vi "get_level.vi"(8 "error in (no error)":errorcluster, 11 "File Log Provider in":refnum<class "File Log Provider.lvclass">) -> (0 "error out":errorcluster, 1 "level":T1 items=["OFF"=0, "FATAL"=100, "ERROR"=200, "WARN"=300, "INFO"=400, "DEBUG"=500, "TRACE"=600, "ALL"=65535], 3 "File Log Provider out":refnum<class "File Log Provider.lvclass">)   [LabVIEW 2019, in "File Log Provider.lvclass"]
uses:
  File Log Provider.lvclass
  Queue Log Provider/Queue Log Provider.lvclass
  Log Service/public/level.ctl
  Log Service/Log Service.lvclass
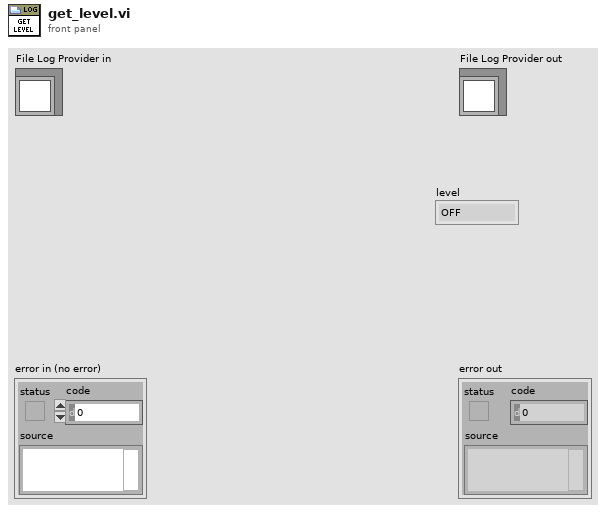
[diagram p1: front panel]
types:
  T1 = typedef "Utility API.lvlib/Log Service.lvclass/level.ctl" = u16
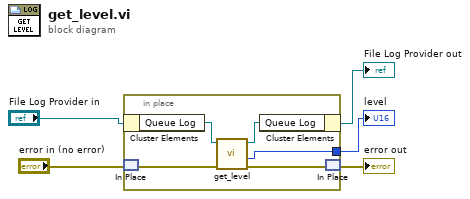
[diagram p0: block diagram]
diagram:
  n1 = in-place {
    in-place-border: [w8] -> w2
    n2 = in-place-cluster #1("File Log Provider in") -> ("Queue Log"=w10:refnum<class "Queue Log Provider.lvclass">)
    n3 = in-place-match #2("error in (no error)") -> (w7:errorcluster)
    n4 = call-dynamic "get_level.vi"("error in (no error)"=w7, "Queue Log Provider in"=w10) -> ("error out"=w6:errorcluster, "level"=w8:T1, "Queue Log Provider out"=w9:refnum<class "Queue Log Provider.lvclass">)  [unwired: 7 in]
    n5 = in-place-cluster #1("Queue Log"=w9) -> (→"File Log Provider out":refnum<class "File Log Provider.lvclass">)
    n6 = in-place-match #2(w6) -> (→"error out":errorcluster)
  }
  "level" <- w2
